vi "New SequenceFile.vi"(8 "error in (no error)":errorcluster, 11 "Engine in":refnum<class "Engine.lvclass">) -> (0 "error out":errorcluster, 2 "New SequenceFile":refnum<class "SequenceFile.lvclass">, 3 "Engine out":refnum<class "Engine.lvclass">)   [LabVIEW 2020, in "TSnax.lvlib" / "Engine.lvclass"]
uses:
  Engine.lvclass
  SequenceFile/SequenceFile.lvclass
  New SequenceFile Request.ctl
  SequenceFile Response.ctl
  Engine.lvclass/Engine.ctl
  9fe03791-84db-4674-9abf-0d5723e09530.vi
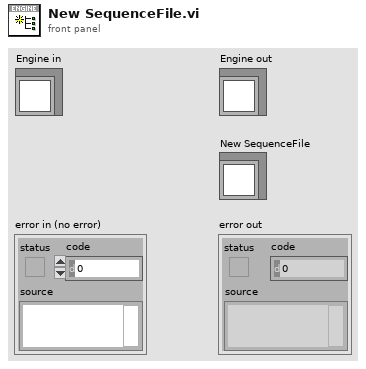
[diagram p1: front panel]
types:
  T1 = typedef "TSnax.lvlib/Engine.lvclass/SequenceFile Response.ctl" = cluster{"SequenceFile":refnum<class "SequenceFile.lvclass">, "Error":errorcluster}
  T2 = typedef "TSnax.lvlib/Engine.lvclass/New SequenceFile Request.ctl" = cluster{"Notifier":refnum<notifier>}
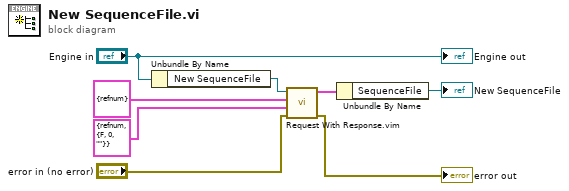
[diagram p0: block diagram]
diagram:
  n1 = Unbundle By Name("Engine in") -> ("New SequenceFile"=w7:refnum<user-event>)
  n2 = call "Request With Response.vim"("error in (no error)"="error in (no error)", "Response Default"=T1 {"SequenceFile"=refnum, "Error"={"status"=FALSE, "code"=0, "source"=""}} ("Open SequenceFile Response"), "Request Data"=T2 {"Notifier"=refnum} ("event data"), "Event"=w7) -> ("error out"=→"error out":errorcluster, "Response"=w3:T1)  [unwired: 6 in]
  n3 = Unbundle By Name(w3) -> ("SequenceFile"=→"New SequenceFile":refnum<class "SequenceFile.lvclass">)
  "Engine out" <- "Engine in"
